vi "Ansteuerung_Frequenzgenerator.vi"(7 "Error_in":errorcluster, 9 "Eingangs-String":string, 10 "VISA-Ressourcenname":refnum<visa-resource-name>="USB0::0x0957::0x0407::MY44043889::INSTR") -> (0 "Error_out":errorcluster, 2 "HardwareAntwort":string, 3 "VISA-Ressourcenname out":refnum<visa-resource-name>="USB0::0x0957::0x0407::MY44043889::INSTR")   [LabVIEW 2016]
doc: "Das VI übergibt der Hardware einen String mit dem Einstellungen gesetzt oder abgefragt werden können."
panel:
  out "Ausgangs String":string
  out "String Länge":dbl
  out "Verbleibender String":string
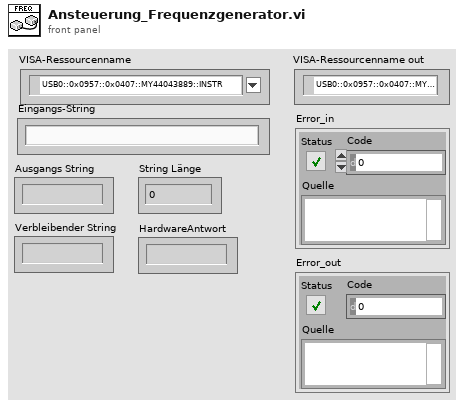
[diagram p1: front panel]
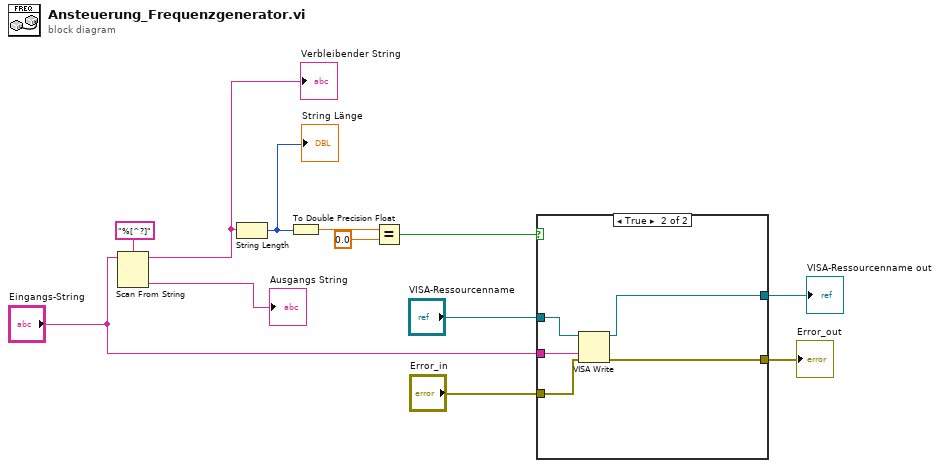
[diagram p0: block diagram]
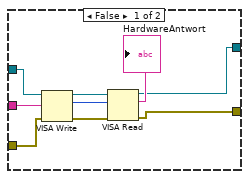
[diagram p2: hidden frame]
diagram:
  n1 = Scan From String(format string="%[^?]" ("Format-String"), input string="Eingangs-String") -> (remaining string=w11:string, output 1=→"Ausgangs String":string)  [unwired: 3 in, 2 out]
  "Verbleibender String" <- w11
  n2 = String Length(string=w11) -> (length=w10:i32)
  "String Länge" <- w10
  n3 = To Double Precision Float(number=w10) -> (double precision float=w8:dbl)
  n4 = Equal?(x=w8, y=0.0) -> (x = y?=w7:bool)
  n5 = case shown="True" w7 {
    tunnel: "Eingangs-String" -> [w18 w26]
    tunnel: "VISA-Ressourcenname" -> [w16 w25]
    tunnel: "Error_in" -> [w15 w24]
    tunnel: [w14 w23] -> w3
    tunnel: [w13 w22] -> w1
    frame False {
      n6 = VISA Write(VISA resource name=w16, write buffer=w18, error in (no error)=w15) -> (VISA resource name out=w20:refnum<visa-resource-name>, return count=w21:u32, error out=w19:errorcluster)
      n7 = VISA Read(VISA resource name=w20, byte count=w21, error in (no error)=w19) -> (VISA resource name out=w13:refnum<visa-resource-name>, read buffer=→"HardwareAntwort":string, error out=w14:errorcluster)  [unwired: 1 out]
    }
    frame True {
      n8 = VISA Write(VISA resource name=w25, write buffer=w26, error in (no error)=w24) -> (VISA resource name out=w22:refnum<visa-resource-name>, error out=w23:errorcluster)  [unwired: 1 out]
    }
  }
  "Error_out" <- w3
  "VISA-Ressourcenname out" <- w1
